vi "open.vi"(8 "error in":errorcluster, 11 "IP Address":string="192.168.0.28") -> (0 "error out":errorcluster, 2 "Identification":string, 3 "TCP":refnum<k5>)   [LabVIEW 2025, in "Newtons4thEkg.lvlib"]
uses:
  Newtons4thEkg.lvlib
  <vilib>/Utility/error.llb/Error Cluster From Error Code.vi
  <vilib>/ErrorRing/Error Ring.xnode
panel:
  # "Newtons4th V0.10\nOpen"
  # "05.05.2025"
  # "Blaz Kelbl"
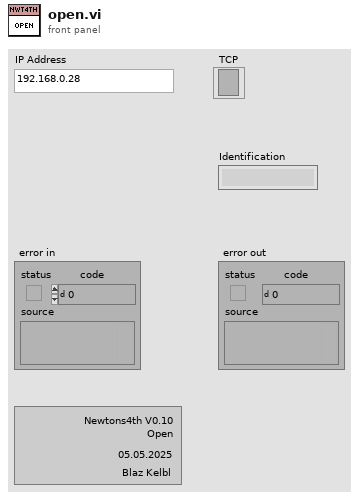
[diagram p1: front panel]
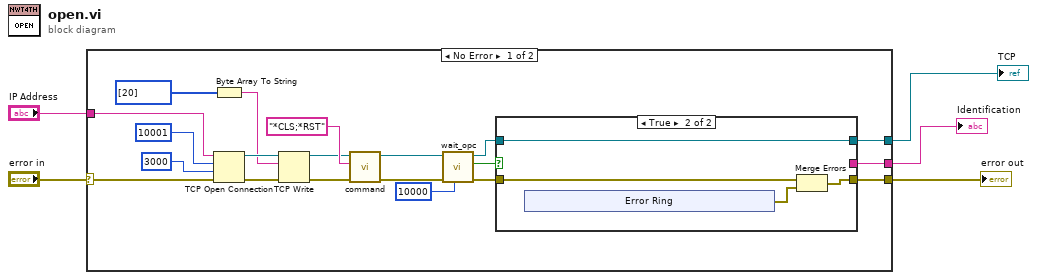
[diagram p0: block diagram]
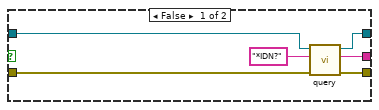
[diagram p2: hidden frame]
diagram:
  n1 = case shown="No Error" "error in" {
    selector: "error in" -> [w24 w41]
    tunnel: "IP Address" -> [w25 _]
    tunnel: [w19 w41] -> w3
    tunnel: [w18 _] -> w2
    tunnel: [w17 _] -> w1
    frame No Error {
      n2 = Byte Array To String(unsigned byte array=u8[] [20]) -> (string=w12:string)
      n3 = TCP Open Connection(address=w25, remote port or service name=u16 10001, timeout ms (60000)=3000, error in (no error)=w24) -> (connection ID=w15:refnum<k5>, error out=w23:errorcluster)  [unwired: 1 in]
      n4 = TCP Write(connection ID=w15, data in=w12, error in (no error)=w23) -> (connection ID out=w14:refnum<k5>, error out=w16:errorcluster)  [unwired: 1 in, 1 out]
      n5 = call "command.vi"("error in (no error)"=w16, "Query"="*CLS;*RST", "TCP in"=w14) -> ("error out"=w11:errorcluster, "TCP out"=w9:refnum<k5>)  [unwired: 7 in]
      n6 = call "wait_opc.vi"("timeout ms (1000)"=10000, "error in (no error)"=w11, "TCP in"=w9) -> ("error out"=w10:errorcluster, "Timeout"=w6:bool, "TCP out"=w8:refnum<k5>)  [unwired: 6 in]
      n7 = case shown="True" w6 {
        tunnel: [w31 w34] -> w19
        tunnel: [w30 w32] -> w18
        tunnel: [w28 _] -> w17
        tunnel: w10 -> [w27 w35]
        tunnel: w8 -> [w26 w32]
        frame False {
          n8 = call "query.vi"("error in (no error)"=w27, "Query"="*IDN?", "TCP in"=w26) -> ("error out"=w31:errorcluster, "Return String"=w28:string, "TCP out"=w30:refnum<k5>)  [unwired: 6 in]
        }
        frame True {
          n9 = xnode "Error Ring"() -> ("error out"=w33:errorcluster)
          n10 = Merge Errors(w35, w33) -> (w34:errorcluster)
        }
      }
    }
    frame Error {
    }
  }
  "error out" <- w3
  "TCP" <- w2
  "Identification" <- w1
